vi "DriveForSpeedDistance.vi"(8 "error in (no error)":errorcluster, 9 "RobotDriveRef":T1={"RobotDriveDevRef"={"DevStatus"={"status"=FALSE, "code"=0, "source"=""}, "Motors[]"=[], "Square Inputs"=FALSE, "Max Output"=0.0}, "Control Mode"=enum."Percent VBus", "Motor Settings"={"Wheel Radius"=0.0, "Encoder Ticks Per Rev"=0.0, "Gear Ratio"=0.0, "ClimbRev"=0.0}, "Default Control Mode"=enum."Unchanged / Invalid", "Speed Mag"=0.0}, 10 "SubSystem Data":T10, 11 "Command Loop Data":cluster{"Start Time (ms)":u32, "Iterations":i32}) -> (0 "error out":errorcluster, 1 "RobotDriveRef Out":T1={"RobotDriveDevRef"={"DevStatus"={"status"=FALSE, "code"=0, "source"=""}, "Motors[]"=[], "Square Inputs"=FALSE, "Max Output"=0.0}, "Control Mode"=enum."Percent VBus", "Motor Settings"={"Wheel Radius"=0.0, "Encoder Ticks Per Rev"=0.0, "Gear Ratio"=0.0, "ClimbRev"=0.0}, "Default Control Mode"=enum."Unchanged / Invalid", "Speed Mag"=0.0}, 2 "Finished":bool, 3 "Left Setpoint":dbl, 4 "Wait Time":dbl, 5 "Right Setpoint":dbl)   [LabVIEW 2015]
uses:
  Drive Setpoints.ctl
  Drive Operations.ctl
  Advanced Drive VIs/RobotDrive Type Def.ctl
  <vilib>/Rock Robotics/WPI/MotorControl/WPI_MotorControlDeviceRef.ctl
  <vilib>/Rock Robotics/WPI/MotorControl/WPI_MotorControlType.ctl
  <vilib>/Rock Robotics/SystemInterfaces/DIO/FPGA_DIOPWMChannel.ctl
  <vilib>/Rock Robotics/WPI/PWM/WPI_PWMDeadband.ctl
  <vilib>/Rock Robotics/WPI/CAN/Jaguar/SubVIs/WPI_CANJaguar_ControlMode.ctl
  <vilib>/Rock Robotics/WPI/CAN/TalonSRX/WPI_CANTalonSRX_APIControlMode.ctl
  Advanced Drive VIs/Drive Motor Settings.ctl
  NavX/NavX Global.vi
  Autonomous/Autonomous Global.vi
  NavX/Library/navX Library v2.lvlib
panel:
  out "Waveform Chart 2":cluster{dbl}(graph)
  out "Waveform Chart":cluster{"Ticks":dbl, "Encoder Position":dbl}(graph)
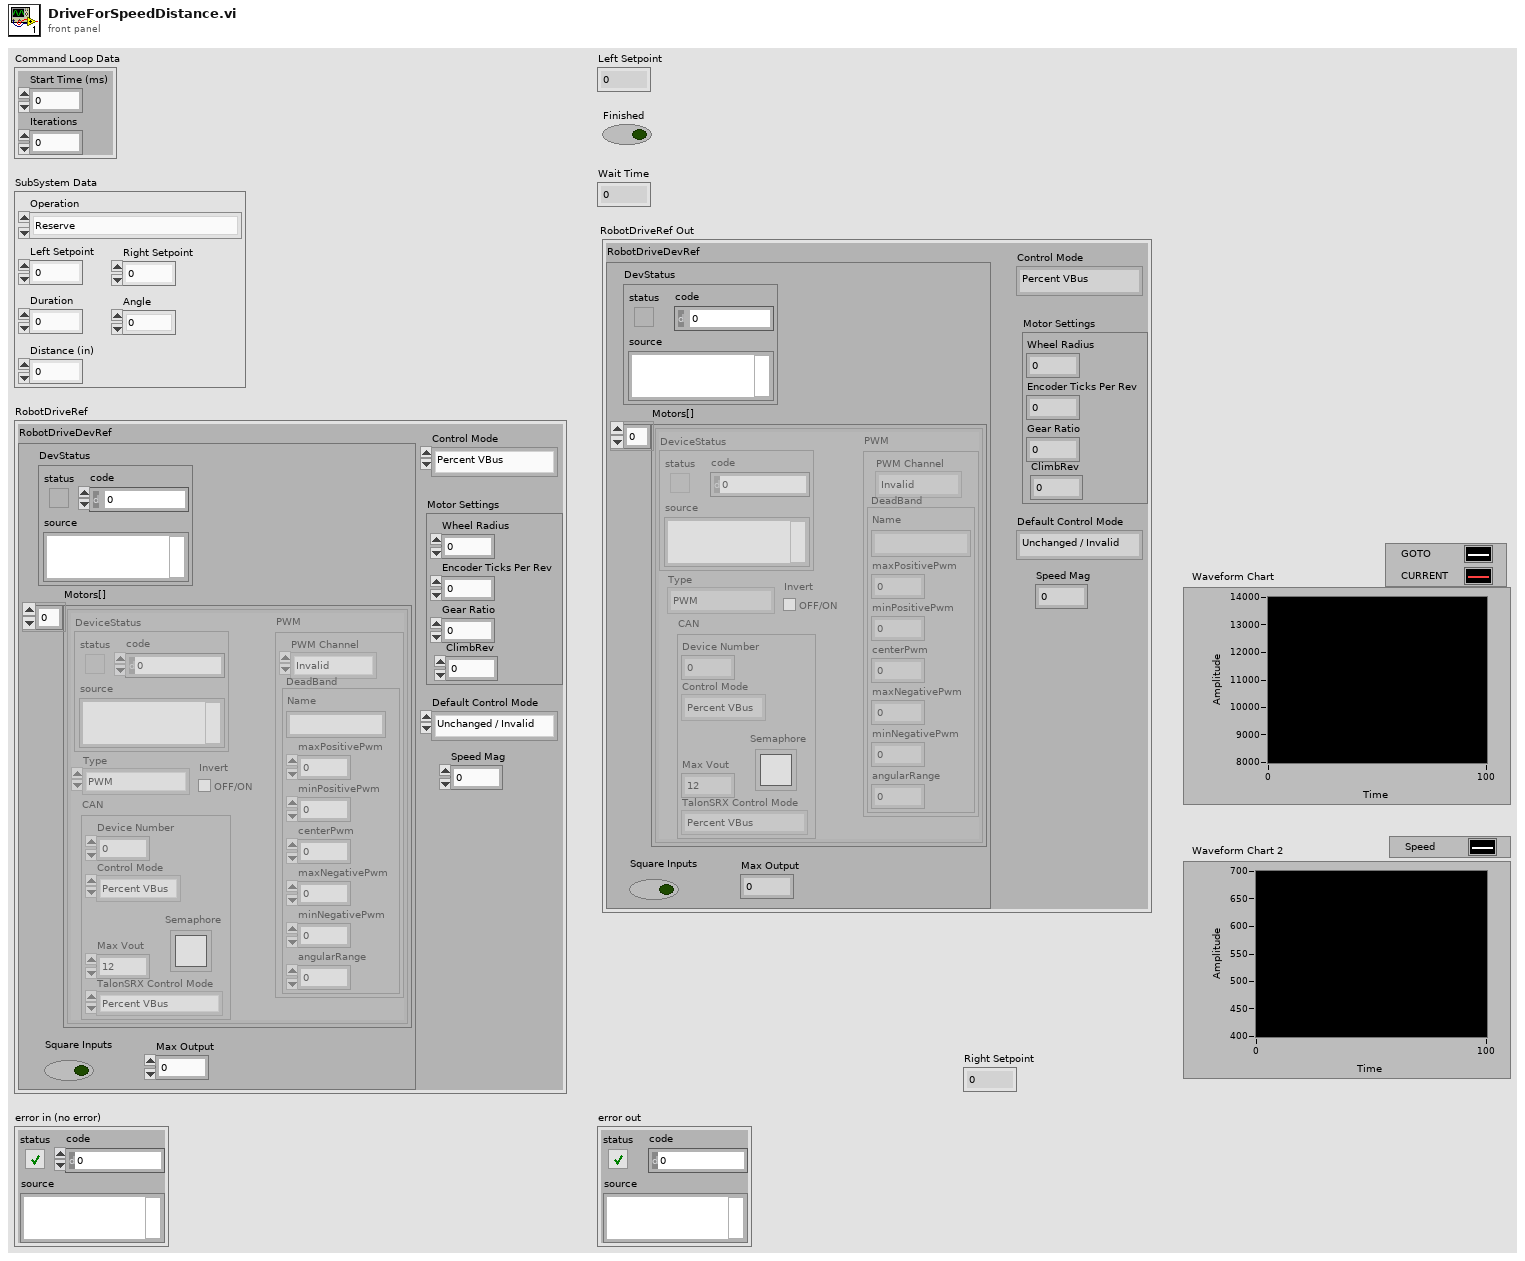
[diagram p1: front panel]
types:
  T1 = typedef "RobotDrive Type Def.ctl" = cluster{"RobotDriveDevRef":cluster{"DevStatus":errorcluster, "Motors[]":T2[], "Square Inputs":bool, "Max Output":dbl}, "Control Mode":T8, "Motor Settings":T9, "Default Control Mode":T8, "Speed Mag":dbl}
  T2 = typedef "WPI_MotorControlDeviceRef.ctl" = cluster{"DeviceStatus":errorcluster, "Type":T3, "PWM":cluster{"PWM Channel":T4, "DeadBand":T5}, "CAN":cluster{"Device Number":u8, "Control Mode":T6, "Semaphore":T7, "Max Vout":dbl, "TalonSRX Control Mode":T8}, "Invert":bool}
  T3 = typedef "WPI_MotorControlType.ctl" = enum16{"PWM", "CAN", "CANTalonSRX"}
  T4 = typedef "FPGA_DIOPWMChannel.ctl" = enum8{"PWM 0", "PWM 1", "PWM 2", "PWM 3", "PWM 4", "PWM 5", "PWM 6", "PWM 7", "PWM 8", "PWM 9", "PWM MXP 0", "PWM MXP 1", "PWM MXP 2", "PWM MXP 3", "PWM MXP 4", "PWM MXP 5", "PWM MXP 6", "PWM MXP 7", "PWM MXP 8", "PWM MXP 9", "Invalid"}
  T5 = typedef "WPI_PWMDeadband.ctl" = cluster{"Name":string, "maxPositivePwm":i32, "minPositivePwm":i32, "centerPwm":i32, "maxNegativePwm":i32, "minNegativePwm":i32, "angularRange":u16}
  T6 = typedef "WPI_CANJaguar_ControlMode.ctl" = enum8{"Percent VBus", "Current", "Speed", "Position", "Voltage"}
  T7 = typedef "Semaphore RefNum" = refnum<k1>
  T8 = typedef "WPI_CANTalonSRX_APIControlMode.ctl" = enum8{"Percent VBus", "Speed", "Position", "Slave", "Unchanged / Invalid", "Voltage Compensation", "Current", "Motion Profile"}
  T9 = typedef "Drive Motor Settings.ctl" = cluster{"Wheel Radius":dbl, "Encoder Ticks Per Rev":dbl, "Gear Ratio":dbl, "ClimbRev":dbl}
  T10 = typedef "Drive Setpoints.ctl" = cluster{"Operation":T11, "Left Setpoint":dbl, "Right Setpoint":dbl, "Duration":dbl, "Angle":dbl, "Distance (in)":dbl}
  T11 = typedef "Drive Operations.ctl" = enum16{"Reserve", "Read Current", "Immediate", "Drive for Time", "Drive for Distance", "Turn Degrees"}
  T12 = typedef "WPI_CANTalonSRX_GlobalStatus.ctl" = cluster{"Applied Throttle":dbl, "Module Enabled":bool, "CAN Error":errorcluster, "Closed Loop Error":dbl, "Forward Limit Switch Closed":bool, "Reverse Limit Switch Closed":bool, "Sensor Position":dbl, "Sensor Velocity":dbl, "Current":dbl, "Sticky Fault - Over Temp":bool, "Sticky Fault - Under Voltage":bool, "Sticky Fault - Forward Limit":bool, "Sticky Fault - Reverse Limit":bool, "Sticky Fault - Forward Soft Limit":bool, "Sticky Fault - Reverse Soft Limit":bool, "Brake is Enabled":bool, "Encoder Position":dbl, "Encoder Velocity":dbl, "Encoder Index Count":dbl, "Encoder A Pin State":bool, "Encoder B Pin State":bool, "Encoder Index Pin State":bool, "Analog In":dbl, "Analog In Velocity":dbl, "Temperature (C)":dbl, "Battery Voltage":dbl, "Control 5 Is Supported":bool, "Current Profile Slot Select":dbl, "Pos Div 8":bool, "Vel Div 4":bool, "Pulse Width Position":i32, "Pulse Width Velocity":i32, "Pulse Width Rise To Rise (us)":i32, "Pulse Width Rise To Fall (us)":i32, "Mot Prof Active Is Under Run":bool, "Mot Prof Active Has Under Run":bool, "Mot Prof Active Is Last":bool, "Mot Prof Active Velocity Only":bool, "Mot Prof Active Is Valid":bool, "Mot Prof Buffer Is Full":bool, "Mot Prof Active Profile Slot Select":i32, "Mot Prof NextID":i32, "Mot Prof Count":i32, "Mot Prof Active Velocity":dbl, "Mot Prof Active Position":dbl, "Mot Prof Output Enable":i32}
  T13 = typedef "navX Library v2.lvlib/Z900_navX_DeviceTypeDef.ctl" = cluster{"Interface":cluster{"Protocol":T14, "Update Rate (4Hz-60Hz)":u8, "navX Open TypeDef":variant}, "Notify Packet":refnum<notifier>, "Loop VI Refnum":refnum<vi>, "Ready to Close Occurrence Refnum":refnum<k4>}
  T14 = typedef "navX Library v2.lvlib/Z900_navX_ProtocolTypeDef.ctl" = enum16{"SERIAL", "I2C", "SPI"}
  T15 = cluster{"Yaw":dbl, "Roll":dbl, "Pitch":dbl, "Heading":dbl, "Fused Heading":dbl}
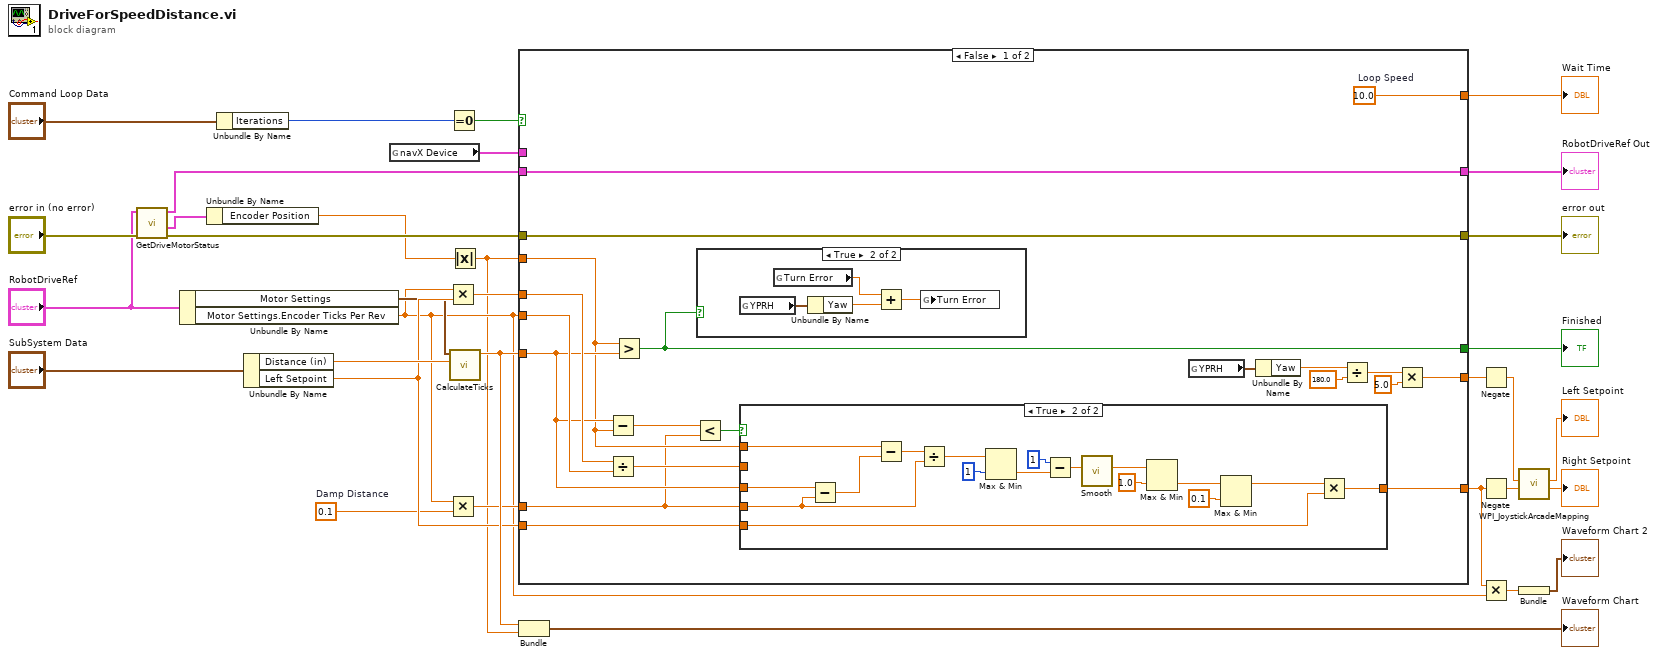
[diagram p0: block diagram]
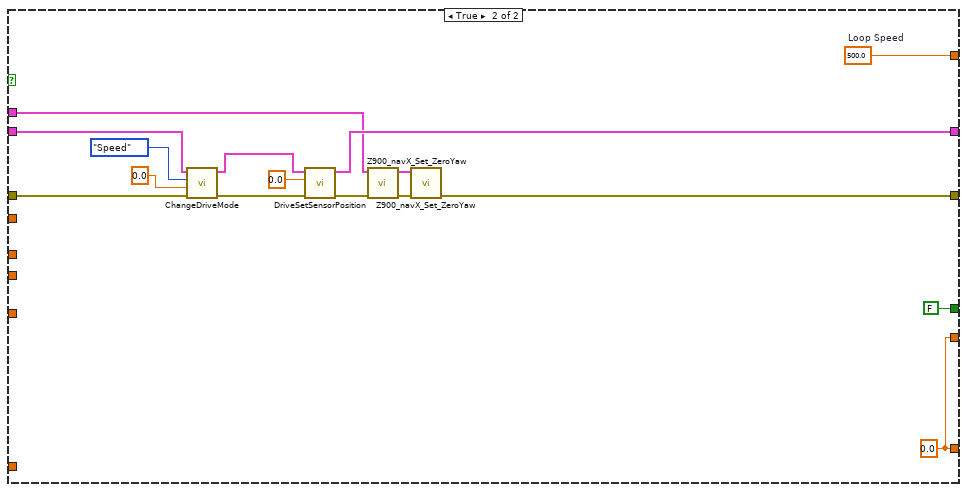
[diagram p4: hidden frame]
diagram:
  w3 = 0.1  # Damp Distance
  n1 = call "GetDriveMotorStatus.vi"("error in (no error)"="error in (no error)", "RobotDriveRef In"="RobotDriveRef") -> ("error out"=w25:errorcluster, "Right"=w22:T12, "RobotDriveRef Out"=w24:T1)  [unwired: 6 in, 1 out]
  n2 = Unbundle By Name("RobotDriveRef") -> ("Motor Settings"=w6:T9, "Motor Settings.Encoder Ticks Per Rev"=w4:dbl)
  n3 = Unbundle By Name(w22) -> ("Encoder Position"=w2:dbl)
  n4 = Unbundle By Name("Command Loop Data") -> ("Iterations"=w31:i32)
  n5 = Unbundle By Name("SubSystem Data") -> ("Distance (in)"=w23:dbl, "Left Setpoint"=w7:dbl)
  n6 = global read "NavX Global.vi" "navX Device"() -> (w19:T13)
  n7 = Multiply(x=w4, y=w7) -> (x*y=w21:dbl)
  n8 = Multiply(x=w4, y=w3) -> (x*y=w5:dbl)
  n9 = Equal To 0?(x=w31) -> (x = 0?=w30:bool)
  n10 = Absolute Value(x=w2) -> (abs(x)=w1:dbl)
  n11 = call "CalculateTicks.vi"("Distance (in)"=w23, "Motor Settings"=w6) -> ("Ticks"=w11:dbl)  [unwired: 9 in]
  n12 = case shown="False" w30 {
    tunnel: [w34 FALSE ("ignore previous (F)")] -> w28
    tunnel: [w39 w77] -> w10
    tunnel: [w53 w85] -> w32
    tunnel: w11 -> [w38 _]
    tunnel: w25 -> [w50 w84]
    tunnel: w24 -> [w53 w83]
    tunnel: w1 -> [w37 _]
    tunnel: w4 -> [w52 _]
    tunnel: w21 -> [w51 _]
    tunnel: [w50 w79] -> w20
    tunnel: w19 -> [_ w78]
    tunnel: [w44 w77] -> w13
    tunnel: [w46 w76] -> w16
    tunnel: w5 -> [w36 _]
    tunnel: w7 -> [w35 _]
    frame False {
      w46 = 10.0  # Loop Speed
      n13 = Subtract(x=w38, y=w37) -> (x-y=w42:dbl)
      n14 = Divide(x=w51, y=w52) -> (x/y=w40:dbl)
      n15 = Greater?(x=w37, y=w38) -> (0:w34:bool)
      n16 = Less?(x=w42, y=w36) -> (x < y?=w41:bool)
      n17 = case shown="True" w34 {
        frame False {
        }
        frame True {
          n18 = global read "NavX Global.vi" "YPRH"() -> (w57:T15)
          n19 = global read "Autonomous Global.vi" "Turn Error"() -> (w55:dbl)
          n20 = Unbundle By Name(w57) -> ("Yaw"=w56:dbl)
          n21 = Add(x=w55, y=w56) -> (x+y=w54:dbl)
          n22 = global write "Autonomous Global.vi" "Turn Error"(w54) -> ()
        }
      }
      n23 = case shown="True" w41 {
        tunnel: w40 -> [w58 _]
        tunnel: [w58 w66] -> w39
        tunnel: w38 -> [_ w75]
        tunnel: w36 -> [_ w69]
        tunnel: w37 -> [_ w74]
        tunnel: w35 -> [_ w65]
        frame False {
        }
        frame True {
          n24 = Subtract(x=w75, y=w69) -> (x-y=w73:dbl)
          n25 = Subtract(x=w74, y=w73) -> (x-y=w70:dbl)
          n26 = Divide(x=w70, y=w69) -> (x/y=w63:dbl)
          n27 = Max & Min(x=w63, y=1) -> (min(x,y)=w62:dbl)  [unwired: 1 out]
          n28 = Subtract(x=1, y=w62) -> (x-y=w67:dbl)
          n29 = call "Smooth.vi"("x"=w67) -> ("y"=w72:dbl)  [unwired: 10 in]
          n30 = Max & Min(x=w72, y=1.0) -> (min(x,y)=w61:dbl)  [unwired: 1 out]
          n31 = Max & Min(x=w61, y=0.1) -> (max(x,y)=w59:dbl)  [unwired: 1 out]
          n32 = Multiply(x=w59, y=w65) -> (x*y=w66:dbl)
        }
      }
      n33 = global read "NavX Global.vi" "YPRH"() -> (w49:T15)
      n34 = Unbundle By Name(w49) -> ("Yaw"=w48:dbl)
      n35 = Divide(x=w48, y=180.0) -> (x/y=w45:dbl)
      n36 = Multiply(x=w45, y=5.0 ("Correct Amp")) -> (x*y=w44:dbl)
    }
    frame True {
      w76 = 500.0  # Loop Speed
      w77 = 0.0 ("output")
      n37 = call "ChangeDriveMode.vi"("error in (no error)"=w84, "Output"=0.0, "Control Mode"=WPI_CANTalonSRX_APIControlMode."Speed", "RobotDriveRef"=w83) -> ("error out"=w88:errorcluster, "RobotDriveRef Out"=w89:T1)  [unwired: 6 in]
      n38 = call "DriveSetSensorPosition.vi"("error in (no error)"=w88, "New Sensor Position"=0.0, "RobotDriveRef In"=w89) -> ("error out"=w80:errorcluster, "RobotDriveRef Out"=w85:T1)  [unwired: 7 in]
      n39 = call "Z900_navX_Set_ZeroYaw.vi"("error in (no error)"=w80, "navX Device"=w78) -> ("error out"=w81:errorcluster, "navX Device"=w82:T13)  [unwired: 8 in]
      n40 = call "Z900_navX_Set_ZeroYaw.vi"("error in (no error)"=w81, "navX Device"=w82) -> ("error out"=w79:errorcluster)  [unwired: 8 in, 1 out]
    }
  }
  "error out" <- w20
  "RobotDriveRef Out" <- w32
  "Finished" <- w28
  "Wait Time" <- w16
  n41 = Bundle("Ticks"=w11, w1) -> (→"Waveform Chart":cluster{"Ticks":dbl, dbl})  [unwired: 1 in]
  n42 = Negate(x=w13) -> (-x=w14:dbl)
  n43 = Negate(x=w10) -> (-x=w15:dbl)
  n44 = Multiply(x=w10, y=w4) -> (x*y=w8:dbl)
  n45 = call <vilib>:"WPI_JoystickArcadeMapping.vi"("Y axis value"=w15, "X axis value"=w14) -> ("Right Motor Value"=→"Right Setpoint":dbl, "Left Motor Value"=→"Left Setpoint":dbl)  [unwired: 8 in]
  n46 = Bundle(w8) -> (→"Waveform Chart 2":cluster{dbl})  [unwired: 1 in]
